vi "test12-Message_Event.vi"(8 "error in (no error)":errorcluster, 11 "TestCase in":refnum<class "testcase-CSMGlobalLog.lvclass">) -> (0 "error out":errorcluster, 3 "TestCase out":refnum<class "testcase-CSMGlobalLog.lvclass">)   [LabVIEW 2017, in "testcase-CSMGlobalLog.lvclass"]
uses:
  testcase-CSMGlobalLog.lvclass
  testcase-CSMGlobalLog.lvclass/testcase-CSMGlobalLog.ctl
  src/user.lib/_NEVSTOP/Communicable State Machine(CSM)/_Support/Typedef/_CSM_GlobalLog_MSG.ctl
  src/user.lib/_NEVSTOP/Communicable State Machine(CSM)/_Support/Typedef/_CSM_Response Source Message.ctl
  src/user.lib/_NEVSTOP/Communicable State Machine(CSM)/_Support/Typedef/_CSM_GlobalLog_MSG_TYPE.ctl
  c0dc643a-0362-49fc-99f4-5251266ba5a0.vi
  src/user.lib/_NEVSTOP/Communicable State Machine(CSM)/_Support/GlobalEvent/GEvt-Generate with Rule Check.vi
  src/user.lib/_NEVSTOP/Communicable State Machine(CSM)/AdvanceAPI/CSM - Convert Error to Argument.vi
  src/user.lib/_NEVSTOP/Communicable State Machine(CSM)/AdvanceAPI/CSM - Make String Arguments Safe.vi
  src/user.lib/_NEVSTOP/Communicable State Machine(CSM)/AdvanceAPI/CSM - Keywords.vi
  src/user.lib/_NEVSTOP/Communicable State Machine(CSM)/_Support/GlobalEvent/Cache-GEvt Refs.vi
  src/user.lib/_NEVSTOP/Communicable State Machine(CSM)/_Support/GlobalEvent/LogFilter/LogFilter - Check.vi
  src/user.lib/_NEVSTOP/Communicable State Machine(CSM)/_Support/GlobalEvent/LogFilter/LogFilter.lvclass
  <vilib>/addons/_JKI Toolkits/VI Tester/TestCase.llb/TestCase.lvclass
  src/user.lib/_NEVSTOP/Communicable State Machine(CSM)/Communicable State Machine.lvlib
  C:/Program Files (x86)/National Instruments/LabVIEW 2017/vi.lib/addons/_JKI Toolkits/VI Tester/TestCase.llb/TestCase.lvclass
panel:
  out "String cache each loop":string
  out "error out 2":errorcluster
  out "Timed out":bool[](array[boolean])
  out "LoopCount":i32
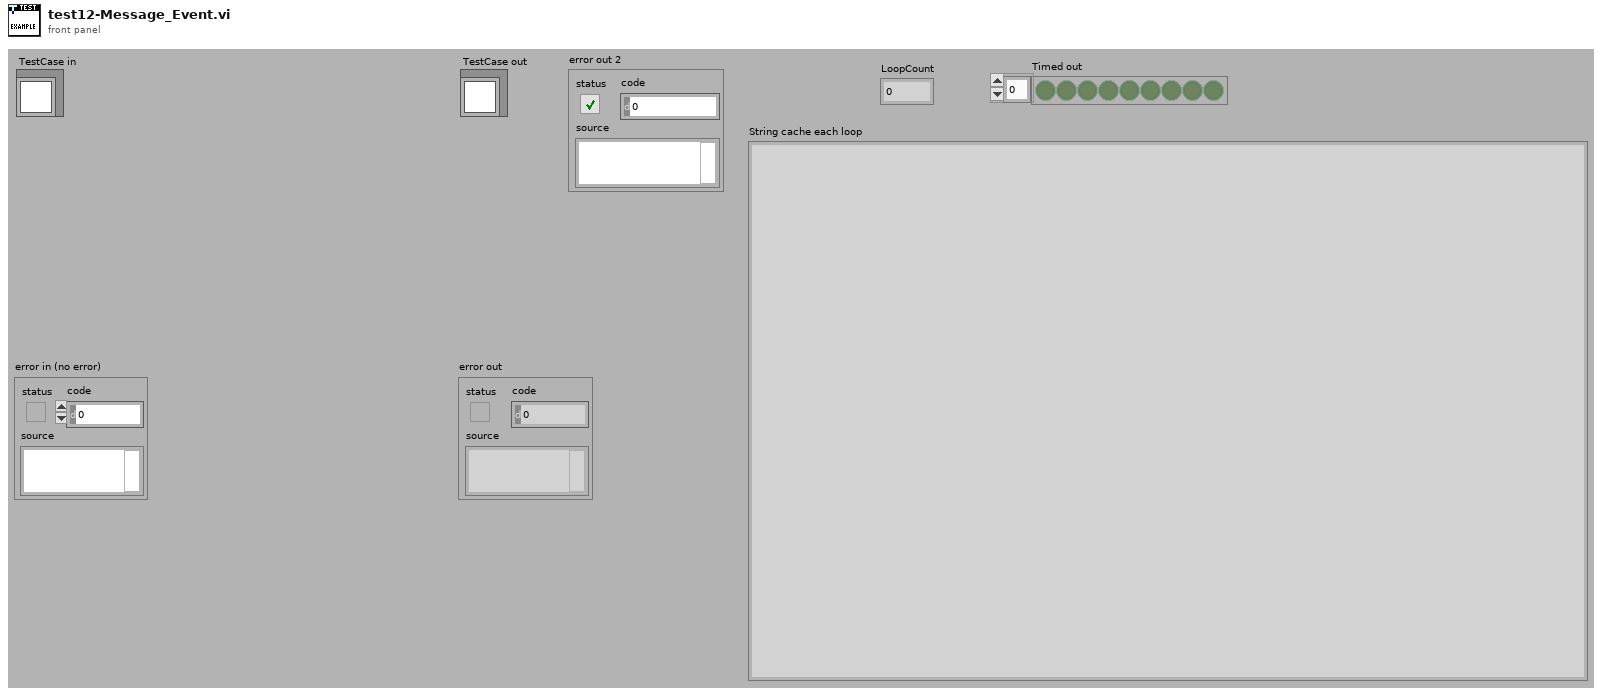
[diagram p1: front panel]
types:
  T1 = typedef "Communicable State Machine.lvlib/_CSM_GlobalLog_MSG.ctl" = cluster{"Name (\"\" to Use UUID)":string, "Current State":string, "Arguments":string, "Source Message":T2, "Source Module":string, "Complete(T)/Start(F)":bool, "LogType":T3, "Time Stamp":timestamp}
  T2 = typedef "Communicable State Machine.lvlib/_CSM_Response Source Message.ctl" = cluster{"‘State":string, "’Arguments":string, "’Error":errorcluster}
  T3 = typedef "Communicable State Machine.lvlib/_CSM_GlobalLog_MSG_TYPE.ctl" = enum16{"User Log", "State Change", "Status", "Interrupt", "Register", "Unregister", "Error Log", "Module Created", "Module Destroyed"}
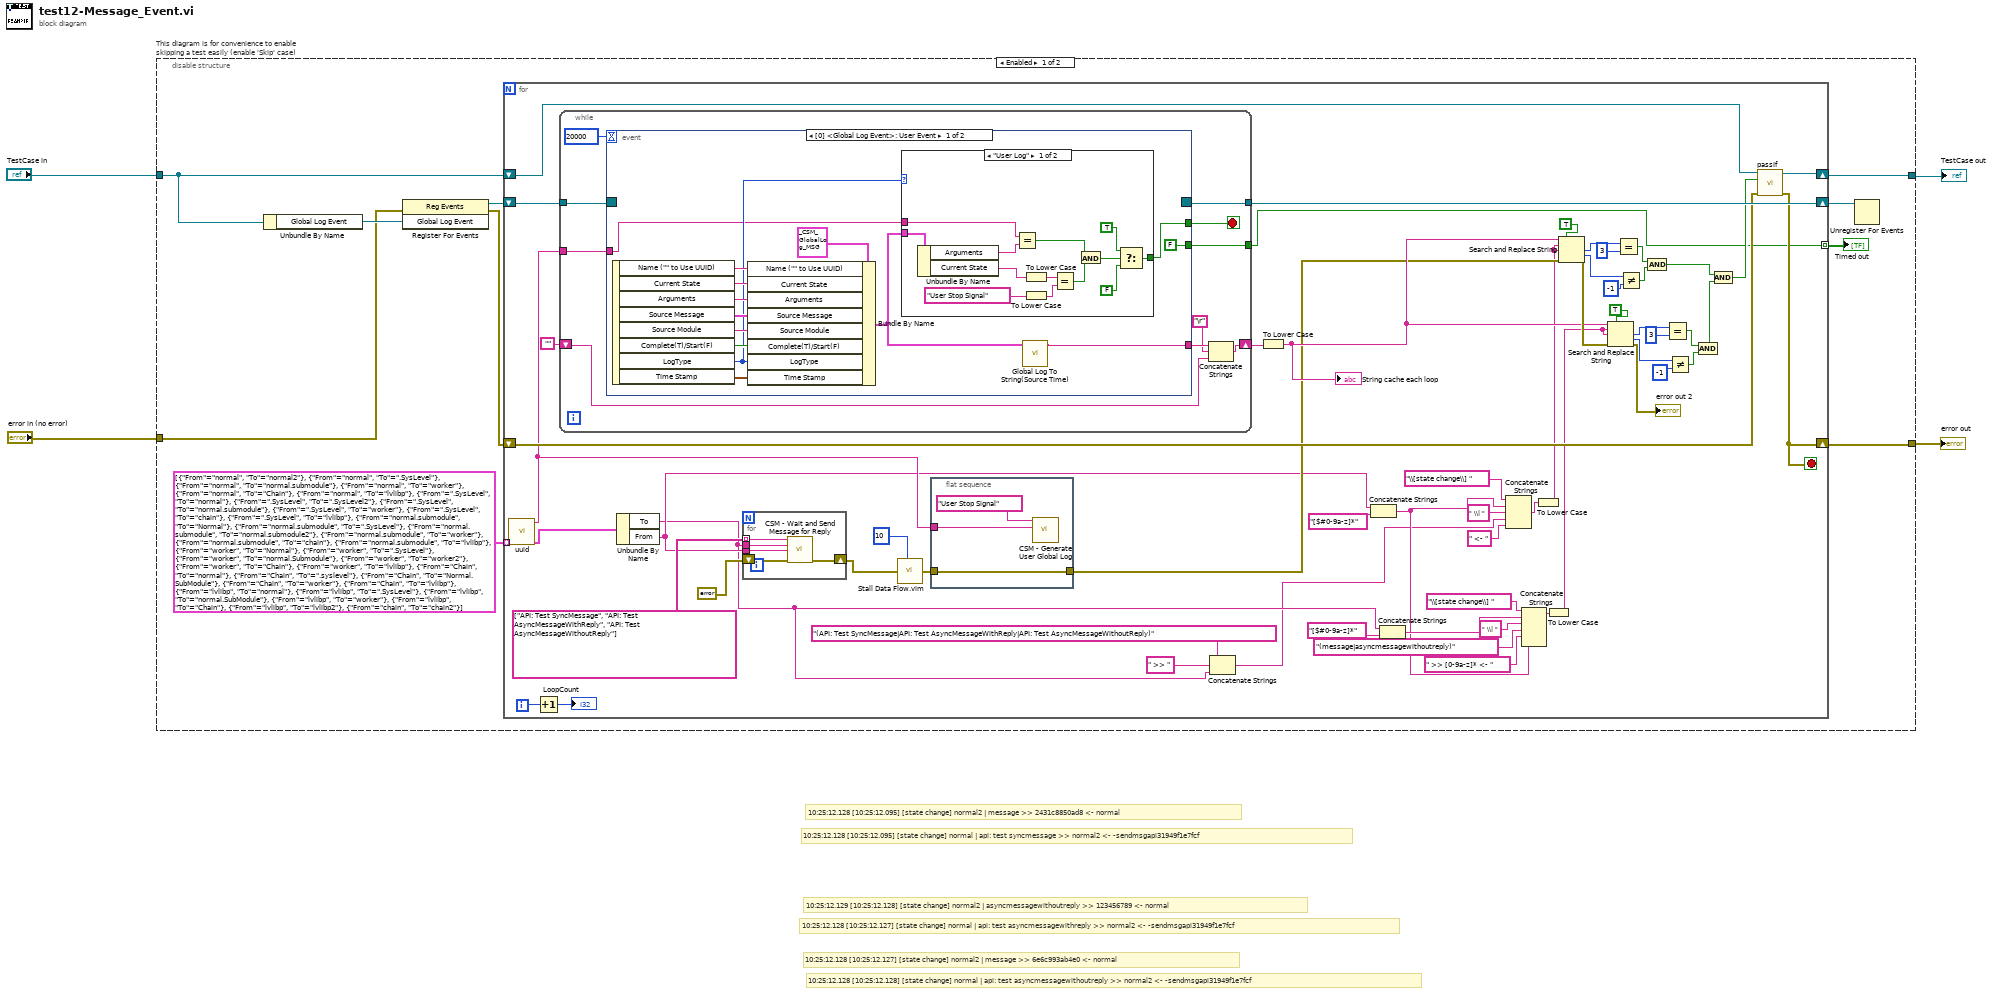
[diagram p0: block diagram]
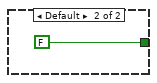
[diagram p2: hidden frame]
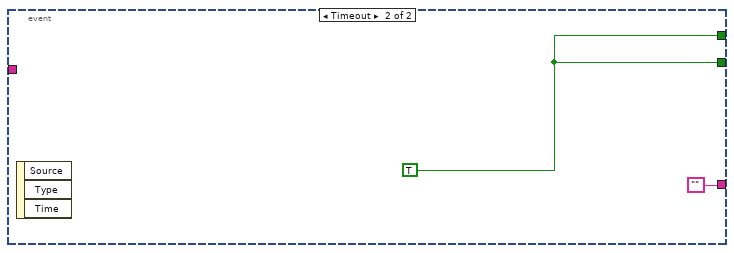
[diagram p3: hidden frame]
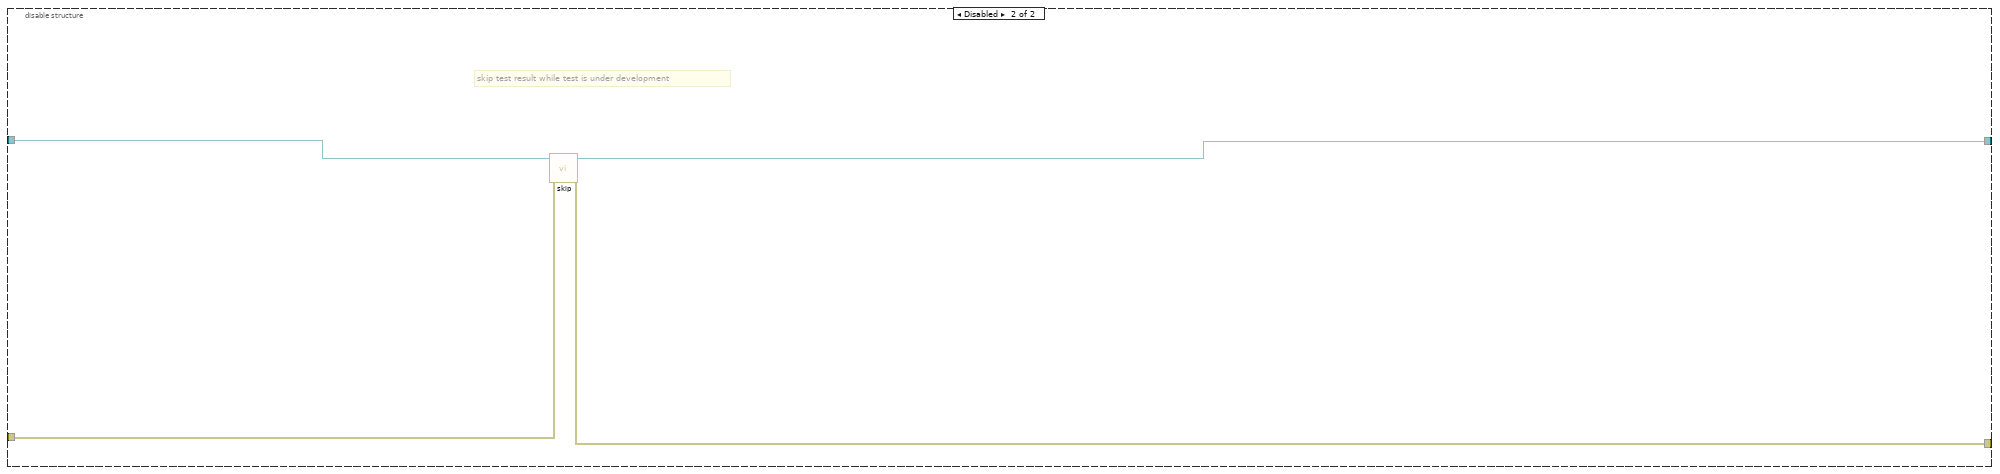
[diagram p4: hidden frame]
diagram:
  # "10:25:12.129 [10:25:12.128] [state change] normal2 | asyncmessagewithoutreply >> 123456789 <- normal"
  # "10:25:12.128 [10:25:12.127] [state change] normal | api: test asyncmessagewithreply >> normal2 <- -sendmsgapi31949f1e7fcf"
  # "10:25:12.128 [10:25:12.127] [state change] normal2 | message >> 6e6c993ab4e0 <- normal"
  # "10:25:12.128 [10:25:12.128] [state change] normal | api: test asyncmessagewithoutreply >> normal2 <- -sendmsgapi31949f1e7fcf"
  # "10:25:12.128 [10:25:12.095] [state change] normal2 | message >> 2431c8850ad8 <- normal"
  # "10:25:12.128 [10:25:12.095] [state change] normal | api: test syncmessage >> normal2 <- -sendmsgapi31949f1e7fcf"
  n1 = disable-structure "This diagram is for convenience to enable skipping a test easily (enable 'Skip' case)" shown="Enabled" {
    disable-tunnel: "TestCase in" -> [w9 w125]
    disable-tunnel: [w8 w123] -> w1
    disable-tunnel: [w7 w124] -> w3
    disable-tunnel: "error in (no error)" -> [w13 w122]
    frame Enabled {
      n2 = Unbundle By Name(w9) -> ("Global Log Event"=w14:refnum<user-event>)
      n3 = register-events(error in=w13, w14) -> (reference out=w12:refnum<event-registration>, error out=w10:errorcluster)  [unwired: 1 in]
      n4 = for {
        shift-right: [w72] -> w11
        shift-left: w12 -> [w73]
        shift-right: [w68] -> w7
        shift-left: w10 -> [w70]
        tunnel: cluster{"From":string, "To":string}[] [{"From"="normal", "To"="normal2"}, {"From"="normal", "To"=".SysLevel"}, {"From"="normal", "To"="normal.submodule"}, {"From"="normal", "To"="worker"}, {"From"="normal", "To"="Chain"}, {"From"="normal", "To"="lvlibp"}, {"From"=".SysLevel", "To"="normal"}, {"From"=".SysLevel", "To"=".SysLevel2"}, {"From"=".SysLevel", "To"="normal.submodule"}, {"From"=".SysLevel", "To"="worker"}, {"From"=".SysLevel", "To"="chain"}, {"From"=".SysLevel", "To"="lvlibp"}, {"From"="normal.submodule", "To"="Normal"}, {"From"="normal.submodule", "To"=".SysLevel"}, {"From"="normal.submodule", "To"="normal.submodule2"}, {"From"="normal.submodule", "To"="worker"}, {"From"="normal.submodule", "To"="chain"}, {"From"="normal.submodule", "To"="lvlibp"}, {"From"="worker", "To"="Normal"}, {"From"="worker", "To"=".SysLevel"}, {"From"="worker", "To"="normal.Submodule"}, {"From"="worker", "To"="worker2"}, {"From"="worker", "To"="Chain"}, {"From"="worker", "To"="lvlibp"}, {"From"="Chain", "To"="normal"}, {"From"="Chain", "To"=".syslevel"}, {"From"="Chain", "To"="Normal.SubModule"}, {"From"="Chain", "To"="worker"}, {"From"="Chain", "To"="lvlibp"}, {"From"="lvlibp", "To"="normal"}, {"From"="lvlibp", "To"=".SysLevel"}, {"From"="lvlibp", "To"="normal.SubModule"}, {"From"="lvlibp", "To"="worker"}, {"From"="lvlibp", "To"="Chain"}, {"From"="lvlibp", "To"="lvlibp2"}, {"From"="chain", "To"="chain2"}] -> [w47] mode=indexing
        shift-right: [w71] -> w8
        shift-left: w9 -> [w67]
        tunnel: [w15] -> w5 mode=indexing
        i -> [w44]
        stop <- w68 stop-if-true
        n5 = call "uuid.vi"() -> ("UUID"=w45:string)  [unwired: 11 in]
        n6 = Increment(x=w44) -> (x+1=→"LoopCount":i32)
        n7 = while {
          tunnel: w73 -> [w91]
          tunnel: [w90] -> w72
          shift-right: [w82] -> w36
          shift-left: "" -> [w85]
          tunnel: w45 -> [w87]
          tunnel: [w86] -> w15
          stop <- w89 stop-if-true
          n8 = event shown="[0] <Global Log Event>: User Event" {
            selector: w91 -> [_ _]
            dyn-events: [_ _] -> w90
            timeout: 20000 -> [_ _]
            tunnel: [w92 ""] -> w84
            tunnel: [w94 w121] -> w89
            tunnel: w87 -> [w95 _]
            tunnel: [FALSE ("Stop") w121] -> w86
            event User Event {
              n9 = event-data() -> ("Name (\"\" to Use UUID)"=w104:string, "Current State"=w103:string, "Arguments"=w102:string, "Source Message"=w101:T2, "Source Module"=w100:string, "Complete(T)/Start(F)"=w99:bool, "LogType"=w96:T3, "Time Stamp"=w98:timestamp)  [unwired: 1 in]
              n10 = Bundle By Name(cluster=T1 {"Name (\"\" to Use UUID)"="", "Current State"="", "Arguments"="", "Source Message"={"‘State"="", "’Arguments"="", "’Error"={"status"=FALSE, "code"=0, "source"=""}}, "Source Module"="", "Complete(T)/Start(F)"=FALSE, "LogType"=enum."State Change", "Time Stamp"=timestamp(0 s since 1904-01-01)} ("Cross CSM Data"), "Name (\"\" to Use UUID)"=w104, "Current State"=w103, "Arguments"=w102, "Source Message"=w101, "Source Module"=w100, "Complete(T)/Start(F)"=w99, "LogType"=w96, "Time Stamp"=w98) -> (w93:T1)
              n11 = case shown="\"User Log\"" w96 {
                tunnel: w93 -> [w118 _]
                tunnel: w95 -> [w117 _]
                tunnel: [w106 FALSE] -> w94
                frame "User Log" {
                  n12 = Unbundle By Name(w118) -> ("Arguments"=w116:string, "Current State"=w115:string)
                  n13 = Equal?(x=w117, y=w116) -> (x = y?=w110:bool)
                  n14 = To Lower Case(string=w115) -> (all lower case string=w114:string)
                  n15 = To Lower Case(string="User Stop Signal" ("Log")) -> (all lower case string=w112:string)
                  n16 = Equal?(x=w114, y=w112) -> (x = y?=w111:bool)
                  n17 = And(x=w110, y=w111) -> (x .and. y?=w109:bool)
                  n18 = Select(t=TRUE, s=w109, f=FALSE) -> (s? t:f=w106:bool)
                }
                frame Default {
                }
              }
              n19 = call "Global Log To String(Source Time).vi"("Log"=w93) -> ("Log String"=w92:string)  [unwired: 9 in]
            }
            event Timeout {
              w121 = TRUE ("Stop")
              n20 = event-data() -> ()  [unwired: 1 in, 3 out]
            }
          }
          n21 = Concatenate Strings(w84, "\r", w85) -> (w82:string)
        }
        n22 = Unbundle By Name(w47) -> ("To"=w19:string, "From"=w23:string)
        n23 = for {
          tunnel: w23 -> [w78]
          tunnel: string[] ["API: Test SyncMessage", "API: Test AsyncMessageWithReply", "API: Test AsyncMessageWithoutReply"] -> [w77] mode=indexing
          tunnel: w19 -> [w76]
          shift-right: [w75] -> w41
          shift-left: errorcluster {"status"=FALSE, "code"=0, "source"=""} ("error out") -> [w74]
          n24 = call "CSM - Wait and Send Message for Reply.vi"("State"=w77, "Arguments (\"\")"=w76, "Target Module"=w78, "Error In (No Error)"=w74) -> ("error out"=w75:errorcluster)  [unwired: 9 in, 2 out]
        }
        n25 = call "Stall Data Flow.vim"("value in"=w41, "milliseconds to wait"=u32 10) -> ("value out"=w46:errorcluster)  [unwired: 1 out]
        n26 = flat-sequence {
          tunnel: w45 -> [w80]
          tunnel: w46 -> [w79]
          tunnel: [w79] -> w37
          frame #0 {
            n27 = call "CSM - Generate User Global Log.vi"("Arguments"=w80, "Log"="User Stop Signal") -> ()  [unwired: 9 in, 1 out]
          }
        }
        n28 = Concatenate Strings("(API: Test SyncMessage|API: Test AsyncMessageWithReply|API: Test AsyncMessageWithoutReply)", " >> " ("string"), w19) -> (w18:string)
        n29 = To Lower Case(string=w36) -> (all lower case string=w38:string)
        "String cache each loop" <- w38
        n30 = Concatenate Strings(w23, "[$#0-9a-z]*" ("string")) -> (w24:string)
        n31 = Concatenate Strings(w19, "[$#0-9a-z]*" ("string")) -> (w25:string)
        n32 = Concatenate Strings("\\[state change\\] " ("regular expression"), w24, " \\| " ("string"), w18, " <- " ("string")) -> (w32:string)
        n33 = Concatenate Strings("\\[state change\\] " ("regular expression"), w25, " \\| " ("string"), "(message|asyncmessagewithoutreply)" ("string"), " >> [0-9a-z]* <- ", w24) -> (w34:string)
        n34 = To Lower Case(string=w32) -> (all lower case string=w17:string)
        n35 = To Lower Case(string=w34) -> (all lower case string=w16:string)
        n36 = Search and Replace String(replace all?=TRUE ("replace all? (F)"), input string=w38, search string=w17, replace string=w17, error in=w37) -> (number of replacements=w55:i32, offset past replacement=w56:i32, error out=w63:errorcluster)  [unwired: 3 in, 1 out]
        n37 = Search and Replace String(replace all?=TRUE ("replace all? (F)"), input string=w38, search string=w16, replace string=w16, error in=w63) -> (number of replacements=w62:i32, offset past replacement=w61:i32, error out=→"error out 2":errorcluster)  [unwired: 3 in, 1 out]
        n38 = Equal?(x=w55, y=3) -> (x = y?=w57:bool)
        n39 = Not Equal?(x=w56, y=-1) -> (x != y?=w58:bool)
        n40 = And(x=w57, y=w58) -> (x .and. y?=w66:bool)
        n41 = Equal?(x=w62, y=3) -> (x = y?=w60:bool)
        n42 = Not Equal?(x=w61, y=-1) -> (x != y?=w59:bool)
        n43 = And(x=w60, y=w59) -> (x .and. y?=w64:bool)
        n44 = And(x=w66, y=w64) -> (x .and. y?=w43:bool)
        n45 = call-dynamic "passIf.vi"("error in (no error)"=w70, "pass"=w43, "TestCase in"=w67) -> ("error out"=w68:errorcluster, "TestCase out"=w71:refnum<class "testcase-CSMGlobalLog.lvclass">)  [unwired: 7 in]
      }
      "Timed out" <- w5
      n46 = Unregister For Events(event registration refnum=w11) -> ()  [unwired: 1 in, 1 out]
    }
    frame Disabled {
      # "skip test result while test is under development"
      n47 = call <vilib>:"skip.vi"("error in (no error)"=w122, "TestCase in"=w125) -> ("error out"=w124:errorcluster, "TestCase out"=w123:refnum<class "testcase-CSMGlobalLog.lvclass">)  [unwired: 8 in]
    }
  }
  "error out" <- w3
  "TestCase out" <- w1
